vi "getRowColor.vi"(0 "reference in":refnum<class "excelFile.lvclass">, 5 "Refnum Cluster In":T1, 9 "End":cluster{"Column":i32, "Row":i32}, 11 "error in (no error)":errorcluster) -> (4 "reference out":refnum<class "excelFile.lvclass">, 15 "error out":errorcluster)   [LabVIEW 2015, in "excelFile.lvclass"]
uses:
  excelFile.lvclass
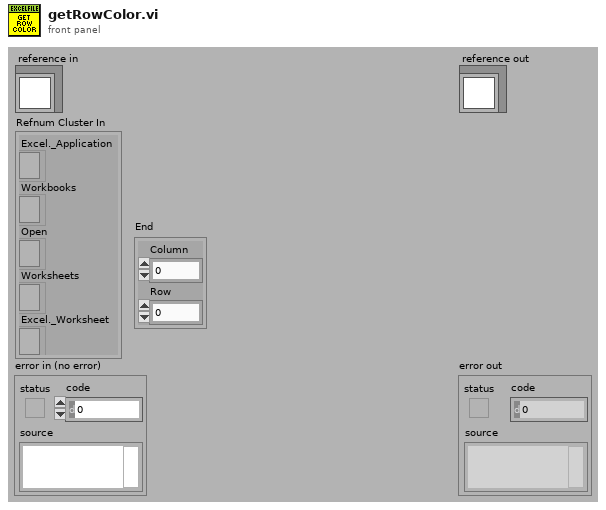
[diagram p1: front panel]
types:
  T1 = cluster{"Excel._Application":refnum<k7>, "Workbooks":refnum<k7>, "Open":refnum<k7>, "Worksheets":refnum<k7>, "Excel._Worksheet":refnum<k7>}
  T2 = typedef "excelFile.lvclass/ObjectAttributesRef.ctl" = refnum<data-value>
  T3 = typedef "excelFile.lvclass/ObjectAttributes.ctl" = cluster{"MyAttribute":dbl, "path":string, "Refnum Excel":cluster{"Excel._Application":refnum<k7>, "Workbooks":refnum<k7>, "Open":refnum<k7>}, "data":string[][][], "save":bool, "fileType":T4, "rowsColor":u32[], "python_ref":refnum<class "python.lvclass">, "items_rows":i32[]}
  T4 = typedef "excelFile.lvclass/fileType.ctl" = enum16{"devices", "items", "partsTracking"}
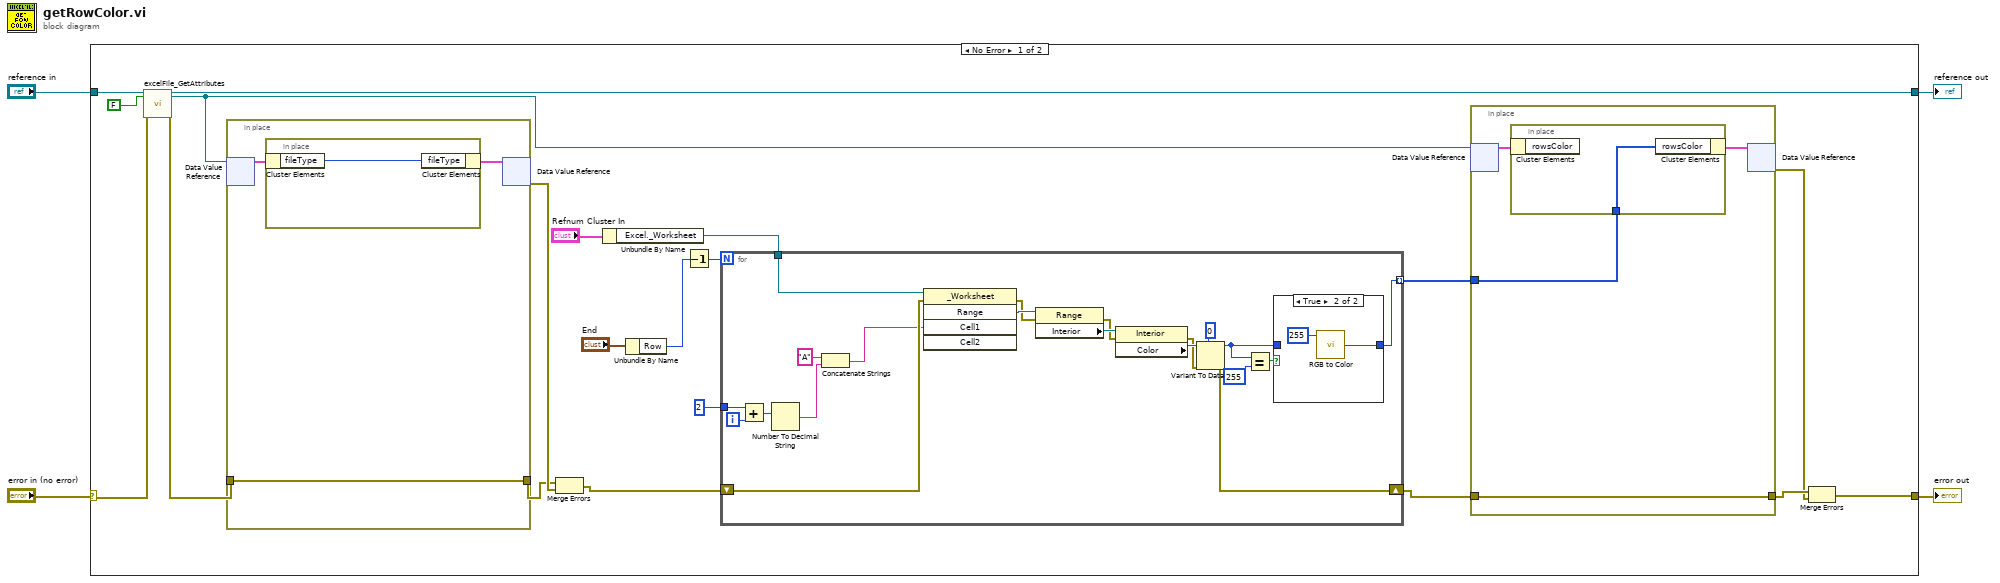
[diagram p0: block diagram]
diagram:
  n1 = case shown="No Error" "error in (no error)" {
    selector: "error in (no error)" -> [w20 w58]
    tunnel: [w7 w58] -> w3
    tunnel: [w18 w57] -> w1
    tunnel: "reference in" -> [w22 w57]
    frame No Error {
      n2 = call "excelFile_GetAttributes.vi"("reference in"=w22, "return data? (T)"=FALSE, "error in (no error)"=w20) -> ("reference out"=w18:refnum<class "excelFile.lvclass">, "attributes ref"=w6:T2, "error out"=w19:errorcluster)  [unwired: 13 in, 1 out]
      n3 = in-place {
        in-place-border: w19 -> [w53]
        in-place-border: [w53] -> w23
        n4 = in-place-dvr #1(w6) -> (w54:T3)  [unwired: 1 out]
        n5 = in-place {
          n6 = in-place-cluster #2(w54) -> ("fileType"=w56:T4)
          n7 = in-place-cluster #2("fileType"=w56) -> (w55:T3)
        }
        n8 = in-place-dvr #1(w55) -> (w24:errorcluster)  [unwired: 1 out]
      }
      n9 = Merge Errors(w23, w24) -> (w14:errorcluster)
      n10 = Unbundle By Name("Refnum Cluster In") -> ("Excel._Worksheet"=w16:refnum<k7>)
      n11 = Unbundle By Name("End") -> ("Row"=w13:i32)
      n12 = Decrement(x=w13) -> (x-1=w12:i32)
      n13 = for {
        N: w12 -> [_]
        tunnel: w16 -> [w42]
        shift-right: [w37] -> w10
        shift-left: w14 -> [w41]
        tunnel: [w31] -> w5 mode=indexing
        tunnel: 2 -> [w34]
        i -> [w36]
        n14 = Add(x=w34, y=w36) -> (x+y=w35:i32)
        n15 = Number To Decimal String(number=w35) -> (decimal integer string=w40:string)  [unwired: 1 in]
        n16 = Concatenate Strings("A" ("string"), w40) -> (w38:string)
        n17 = invoke class="_Worksheet" method="Range"(reference=w42, error in=w41, "Cell1"=w38) -> (error out=w47:errorcluster, "Range"=w49:refnum<k7>)  [unwired: 2 in, 3 out]
        n18 = property class="Range"(reference=w49, error in=w47) -> (error out=w46:errorcluster, "Interior"=w48:refnum<k7>)  [unwired: 1 out]
        n19 = property class="Interior"(reference=w48, error in=w46) -> (error out=w43:errorcluster, "Color"=w45:variant)  [unwired: 1 out]
        n20 = Variant To Data(error in=w43, type=u32 0, Variant=w45) -> (data=w30:u32, error out=w37:errorcluster)
        n21 = Equal?(x=w30, y=u32 255) -> (x = y?=w32:bool)
        n22 = case shown="True" w32 {
          tunnel: [w50 w52] -> w31
          tunnel: w30 -> [w50 _]
          frame False {
          }
          frame True {
            n23 = call <vilib>:"RGB to Color.vi"("R"=u8 255) -> ("Color"=w52:u32)  [unwired: 2 in]
          }
        }
      }
      n24 = in-place {
        in-place-border: w10 -> [w26]
        in-place-border: [w26] -> w9
        in-place-border: w5 -> [w25]
        n25 = in-place-dvr #3(w6) -> (w27:T3)  [unwired: 1 out]
        n26 = in-place {
          in-place-border: w25 -> [w29]
          n27 = in-place-cluster #4(w27) -> ()  [unwired: 1 out]
          n28 = in-place-cluster #4("rowsColor"=w29) -> (w28:T3)
        }
        n29 = in-place-dvr #3(w28) -> (w8:errorcluster)  [unwired: 1 out]
      }
      n30 = Merge Errors(w9, w8) -> (w7:errorcluster)
    }
    frame Error {
    }
  }
  "error out" <- w3
  "reference out" <- w1
